vi "Read Coils.vi"(8 "error in":errorcluster, 9 "number of coils":u16, 10 "starting address":u16, 11 "device data model in":refnum<class "Device Data Model.lvclass">) -> (0 "error out":errorcluster, 2 "data":bool[](array[boolean]), 3 "device data model out":refnum<class "Device Data Model.lvclass">)   [LabVIEW 2012, in "Device Data Model.lvclass"]
doc: "Reads N coils from the data model starting at address M."
uses:
  Device Data Model.lvclass
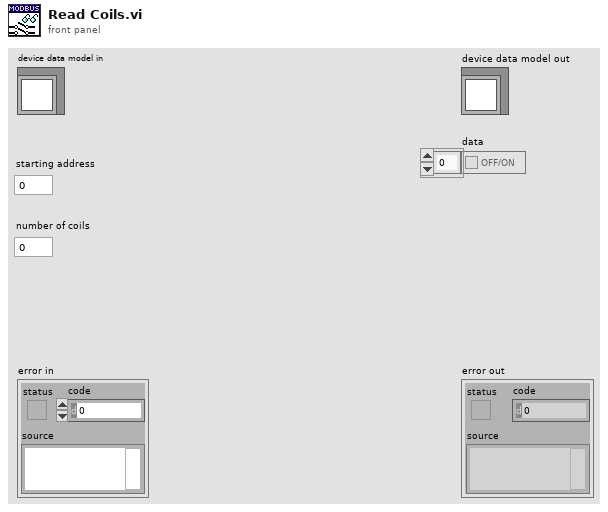
[diagram p1: front panel]
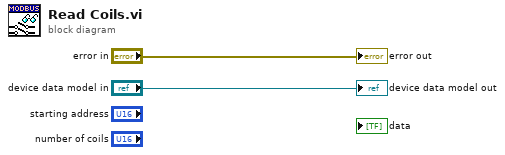
[diagram p0: block diagram]
diagram:
  "error out" <- "error in"
  "device data model out" <- "device data model in"
